vi "Write Construct String Camera Status.lvclass.vi"(8 "error in (no error)":errorcluster, 10 "Construct String Camera Status.lvclass":refnum<class "Construct String Camera Status.lvclass">, 11 "RxTxCamera in":refnum<class "RxTxCamera.lvclass">) -> (0 "error out":errorcluster, 3 "RxTxCamera out":refnum<class "RxTxCamera.lvclass">)   [LabVIEW 2018, in "RxTxCamera.lvclass"]
doc: "Este VI escreve o construtor do status da câmera na classe"
uses:
  RxTxCamera.lvclass
  Construct String Camera Status/Construct String Camera Status.lvclass
  RxTxCamera.lvclass/RxTxCamera.ctl
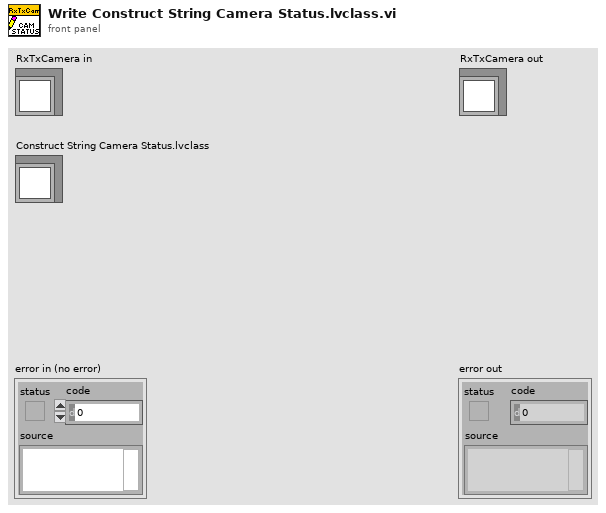
[diagram p1: front panel]
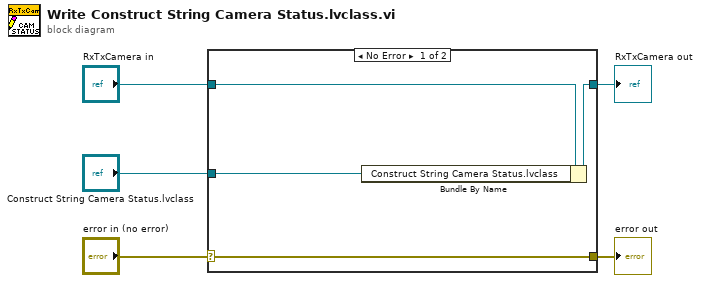
[diagram p0: block diagram]
diagram:
  n1 = case shown="No Error" "error in (no error)" {
    selector: "error in (no error)" -> [w9 w10]
    tunnel: [w9 w10] -> w4
    tunnel: [w7 w11] -> w2
    tunnel: "RxTxCamera in" -> [w8 w11]
    tunnel: "Construct String Camera Status.lvclass" -> [w6 _]
    frame No Error {
      n2 = Bundle By Name(cluster=w8, "Construct String Camera Status.lvclass"=w6) -> (w7:refnum<class "RxTxCamera.lvclass">)
    }
    frame Error {
    }
  }
  "error out" <- w4
  "RxTxCamera out" <- w2
